vi "PlotSpectrum.vi"() -> ()   [LabVIEW 2012]
uses:
  Type/_Peak Property.ctl
panel:
  in  "Search Window":dbl=0.8
  in  "threshold":dbl=1000.0
  out "Peak":T1
  out "Found":bool
  in  "RefMass":dbl=1778.3
  out "Peak List":T1[](array[typedef])
  in  "file path (dialog if empty)":path=path "C:/Users/Min/Projects/SVN/Sniffer900/Server/PeakDetection/Q1 PPG Pos IonSniffer-140926.txt"
  out "time(mS)":u32
  out "# found":i32
  out "XY Graph":cluster{"X":dbl, "Y":dbl}[](graph)
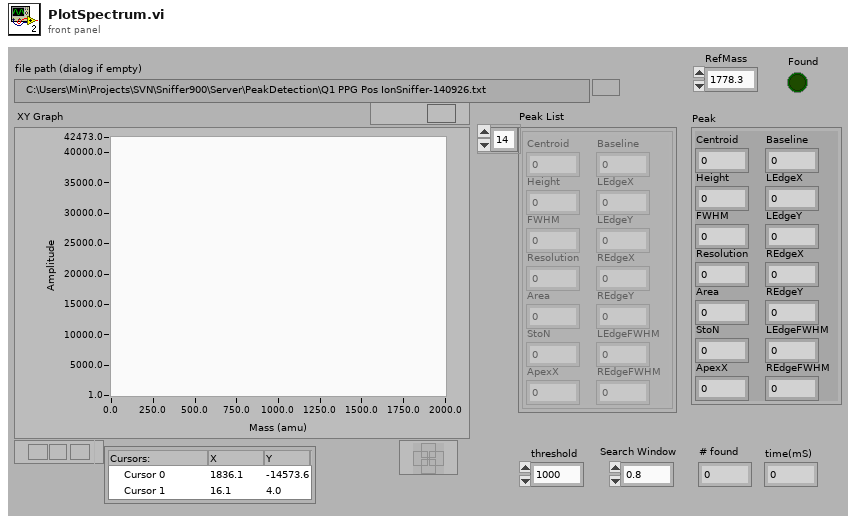
[diagram p1: front panel]
types:
  T1 = typedef "_Peak Property.ctl" = cluster{"Centroid":dbl, "Height":dbl, "FWHM":dbl, "Resolution":dbl, "Area":dbl, "StoN":dbl, "ApexX":dbl, "Baseline":dbl, "LEdgeX":dbl, "LEdgeY":dbl, "REdgeX":dbl, "REdgeY":dbl, "LEdgeFWHM":dbl, "REdgeFWHM":dbl}
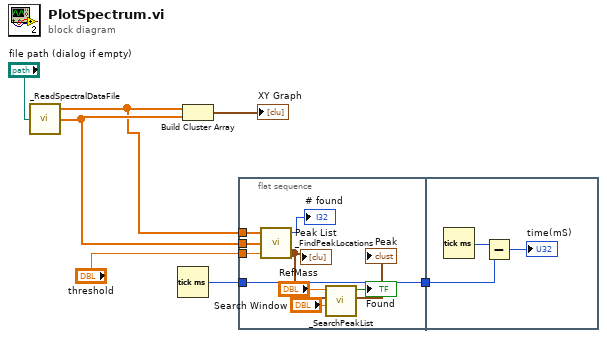
[diagram p0: block diagram]
diagram:
  n1 = call "_ReadSpectralDataFile.vi"("file path (dialog if empty)"="file path (dialog if empty)") -> ("Y"=w6:dbl[], "X"=w4:dbl[])  [unwired: 1 out]
  n2 = Tick Count (ms)() -> (millisecond timer value=w3:u32)
  n3 = Build Cluster Array(w4, w6) -> (→"XY Graph":cluster{dbl, dbl}[])
  n4 = flat-sequence {
    tunnel: w6 -> [w17]
    tunnel: "threshold" -> [w16]
    tunnel: w4 -> [w14]
    tunnel: w3 -> [w13]
    tunnel: [w13] -> w2
    tunnel: w2 -> [w19]
    frame #0 {
      n5 = call "_FindPeakLocations.vi"("threshold"=w16, "Intensities"=w17, "Masses"=w14) -> ("Peak List"=w12:T1[], "# found"=→"# found":i32)  [unwired: 1 in]
      "Peak List" <- w12
      n6 = call "_SearchPeakList.vi"("Search Window (3)"="Search Window", "Peak List"=w12, "RefMass"="RefMass") -> ("Peak"=→"Peak":T1, "Found"=→"Found":bool)  [unwired: 2 in, 1 out]
    }
    frame #1 {
      n7 = Tick Count (ms)() -> (millisecond timer value=w20:u32)
      n8 = Subtract(x=w20, y=w19) -> (x-y=→"time(mS)":u32)
    }
  }
